vi "Create Data File.vi"(8 "Error In":errorcluster, 9 "file name":string="Test Report", 10 "prompt (Create Folder)":string="logs", 11 "base path":path) -> (0 "Error Out":errorcluster, 3 "File Refnum":refnum<file>)   [LabVIEW 2018]
doc: "This VI performs a series of tasks to create a file for logging data:\n\n1) Check to see if a folder called 'Logged Data' exsists in the same directory as the application\n2) If the folder does not exsist, create it\n3) Create a file name of the format 'Acquired Data <Date> <Time>.txt'\n4) Replace or Create the file"
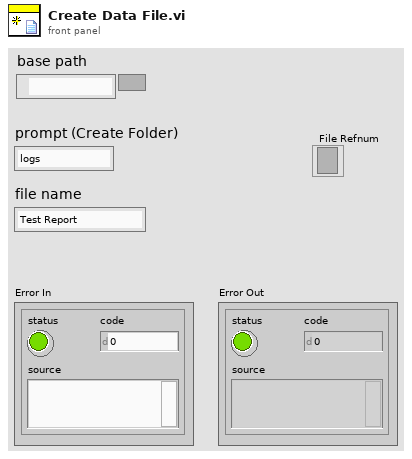
[diagram p1: front panel]
types:
  T1 = enum16{"open", "replace", "create", "open or create", "replace or create", "replace or create with confirmation"}
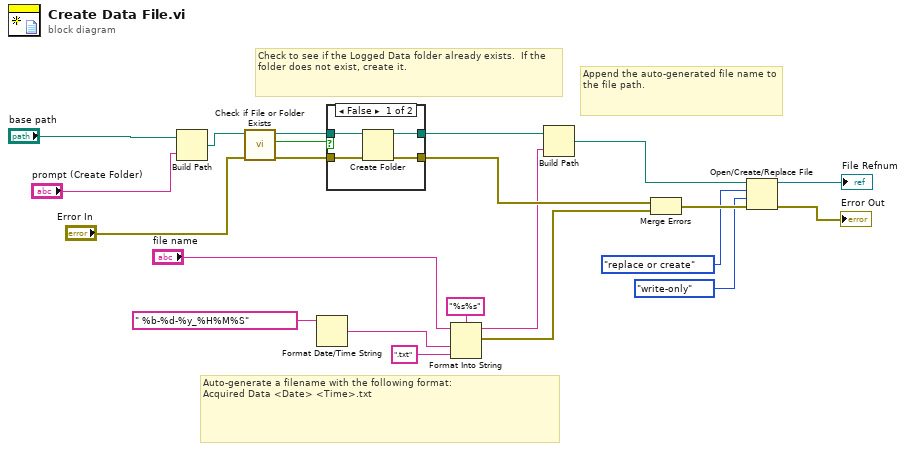
[diagram p0: block diagram]
diagram:
  # "Append the auto-generated file name to the file path."
  # "Check to see if the Logged Data folder already exists.  If the folder does not exist, create it."
  # "Auto-generate a filename with the following format:\nAcquired Data <Date> <Time>.txt"
  n1 = Build Path(base path="base path", name or relative path="prompt (Create Folder)") -> (appended path=w12:path)
  n2 = call <vilib>:"Check if File or Folder Exists.vi"("error in (no error)"="Error In", "path"=w12) -> ("error out"=w11:errorcluster, "file or folder exists?"=w9:bool, "dup path"=w10:path)  [unwired: 7 in]
  n3 = Format Date/Time String(time format string (%c)=" %b-%d-%y_%H%M%S") -> (date/time string=w5:string)  [unwired: 2 in]
  n4 = case shown="False" w9 {
    tunnel: [w26 w28] -> w15
    tunnel: [w25 w27] -> w14
    tunnel: w11 -> [w24 w27]
    tunnel: w10 -> [w23 w28]
    frame False {
      n5 = Create Folder(path (use dialog)=w23, error in=w24) -> (created path=w26:path, error out=w25:errorcluster)  [unwired: 1 in, 1 out]
    }
    frame True {
    }
  }
  n6 = Format Into String(format string="%s%s", initial string="file name", w5, ".txt" ("string")) -> (resulting string=w2:string, error out=w3:errorcluster)  [unwired: 1 in]
  n7 = Build Path(base path=w15, name or relative path=w2) -> (appended path=w22:path)
  n8 = Merge Errors(w14, w3) -> (w21:errorcluster)
  n9 = Open/Create/Replace File(file path (use dialog)=w22, error in=w21, operation (0:open)=T1."replace or create", access (0:read/write)=enum16{"read/write", "read-only", "write-only"}."write-only") -> (refnum out=→"File Refnum":refnum<file>, error out=→"Error Out":errorcluster)  [unwired: 2 in, 1 out]
